vi "T7 Read Cal Constants KAG.vi"(0 "IP:Port":string, 4 "Flash Write Registers":T4(array[cluster])=[{"Register Num"=61800, "Register Name"="INTERNAL_FLASH_KEY", "DataType"="UINT32", "Write Val"=1134709826.0}, {"Register Num"=61810, "Register Name"="INTERNAL_FLASH_READ_POINTER", "DataType"="UINT32", "Write Val"=3948544.0}] {"Write Val" format="%#.0f"}, 5 "Stream Configuration":T2={"Scan Rate (Hz)"=1000.0, "Samples Per Packet"=512, "Resolution Index"=0, "Buffer Size (bytes)"=32768, "NumScans"=1500, "Read Timeout (ms)"=5000, "Scan Table"=[{"Channel"=0, "BipGain"=0, "Input Config"="Single-Ended"}, {"Channel"=1, "BipGain"=0, "Input Config"="Single-Ended"}, {"Channel"=2, "BipGain"=0, "Input Config"="Single-Ended"}, {"Channel"=3, "BipGain"=0, "Input Config"="Single-Ended"}]} {"Samples Per Packet" max=512 step=1; "Buffer Size (bytes)" max=32768 step=1; "Resolution Index" max=8 step=1; "Scan Rate (Hz)" max=100000; "Scan Table"."BipGain" items=["x1", "x10", "x100", "x1000"]; "Scan Table"."Channel" step=1}, 6 "Flash Read Registers":T4(array[cluster])=[{"Register Num"=61812, "Register Name"="INTERNAL_FLASH_READ", "DataType"="UINT32", "Write Val"=0.0}], 7 "Secondary Stream Configurations":T1={"Settling Delay (*5 us)"=0.0, "Clock Source"=0, "Auto Target"=1} {"Auto Target" max=255 step=1; "Clock Source" max=2 step=2; "Settling Delay (*5 us)" min=0 max=5000 step=1}, 11 "error in":errorcluster) -> (8 "Calibration Constants":T5(array[cluster]) {"PSlope" format="%#.13f"; "NSlope" format="%#.13f"; "AvgSlope" format="%#.13f"; "Center" format="%#.13f"; "Offset" format="%#.13f"}, 15 "error out":errorcluster)   [LabVIEW 2022 SP3]
doc: "Write Stream Configuration LabJack Registers via MODBUS. There are a set of registers which comprise the stream configuration registers, and these are written with control values for Scan Rate, NumScans, Resolution, etc. Also, the Scan Table is used to build a Scan List of Stream Configuration Registers which point to streamable AI Channels."
uses:
  T7 Stream Config KAG.ctl
  T7 Secondary Configs KAG.ctl
  T7 Stream Globals KAG.vi
panel:
  in  "Tab Control":T3(tab)=enum."Flash Data"
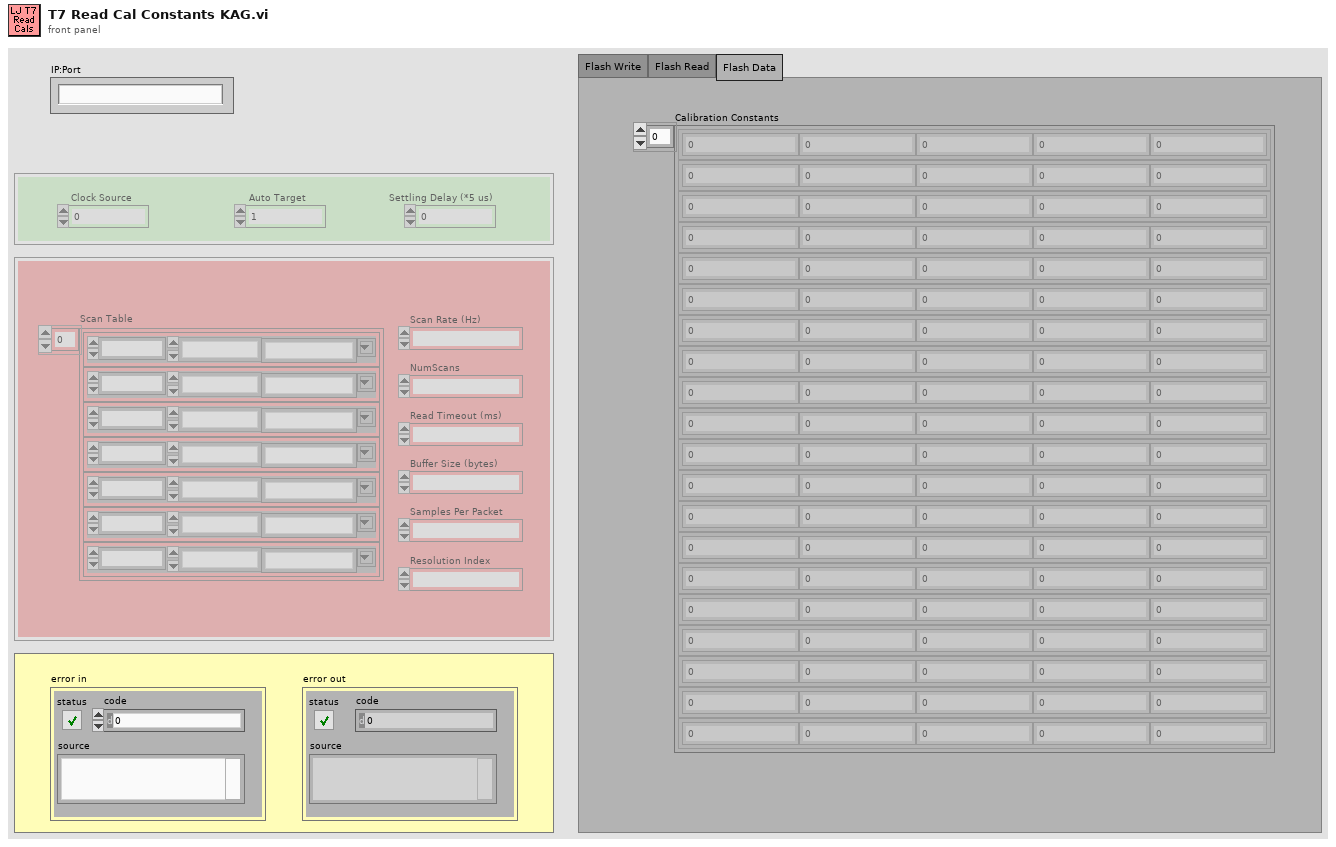
[diagram p1: front panel]
types:
  T1 = typedef "T7 Secondary Configs KAG.ctl" = cluster{"Settling Delay (*5 us)":sgl, "Clock Source":u32, "Auto Target":u32}
  T2 = typedef "T7 Stream Config KAG.ctl" = cluster{"Scan Rate (Hz)":sgl, "Samples Per Packet":u32, "Resolution Index":u32, "Buffer Size (bytes)":u32, "NumScans":u32, "Read Timeout (ms)":u32, "Scan Table":cluster{"Channel":u32, "BipGain":u32, "Input Config":string}[]}
  T3 = enum32{"Flash Write", "Flash Read", "Flash Data"}
  T4 = cluster{"Register Num":i32, "Register Name":string, "DataType":string, "Write Val":dbl}[]
  T5 = cluster{"PSlope":dbl, "NSlope":dbl, "AvgSlope":dbl, "Center":dbl, "Offset":dbl}[]
  T6 = cluster{"Register Num":i32, "Register Name":string, "DataType":string, "Write Val":dbl}
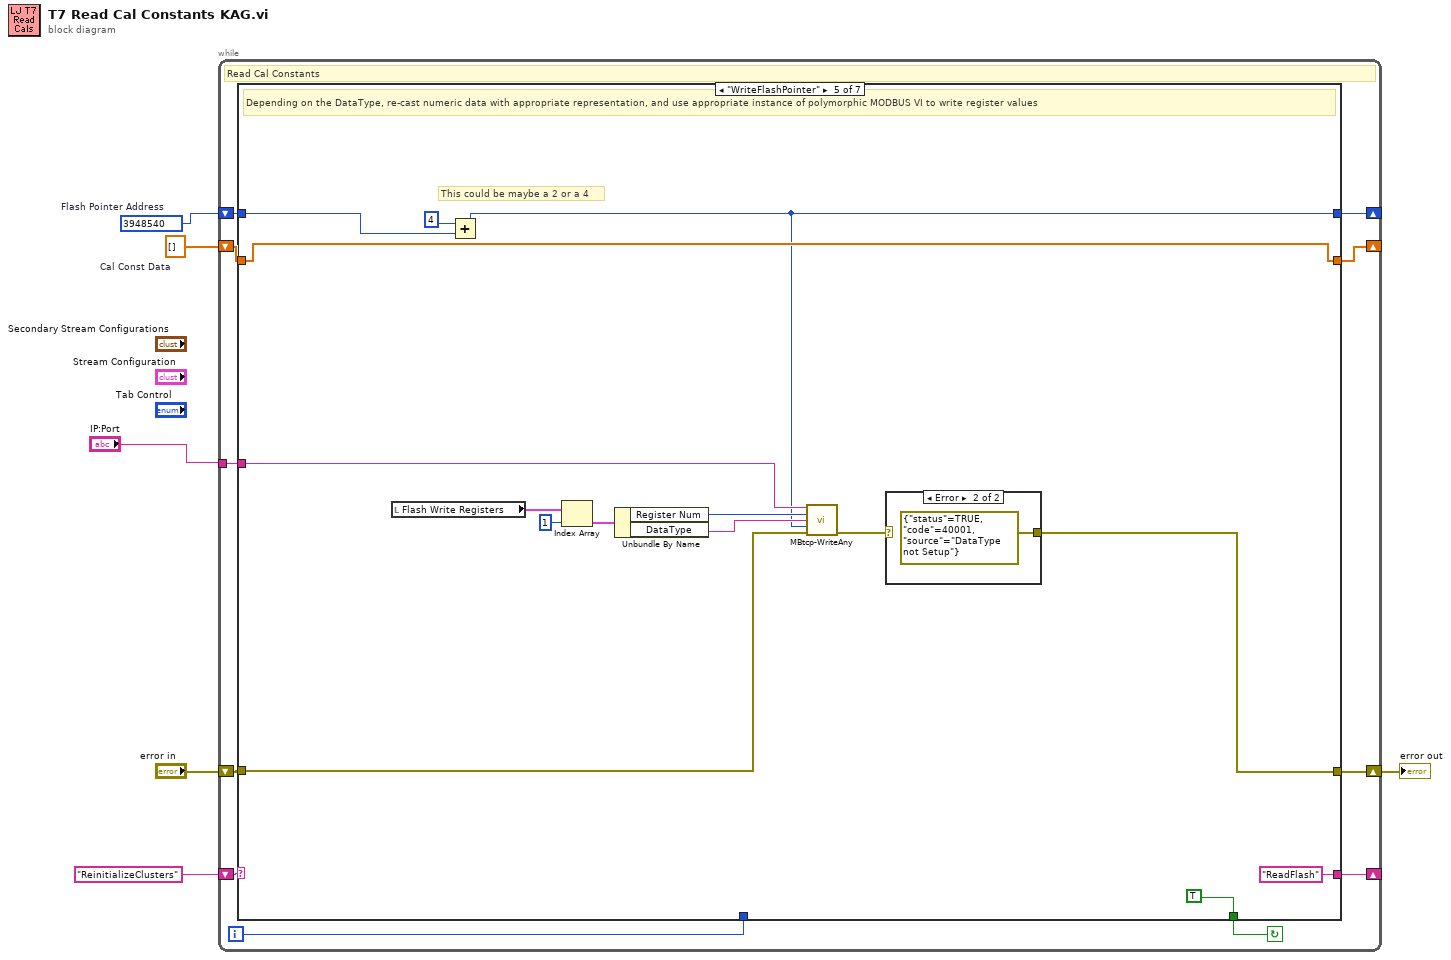
[diagram p0: block diagram]
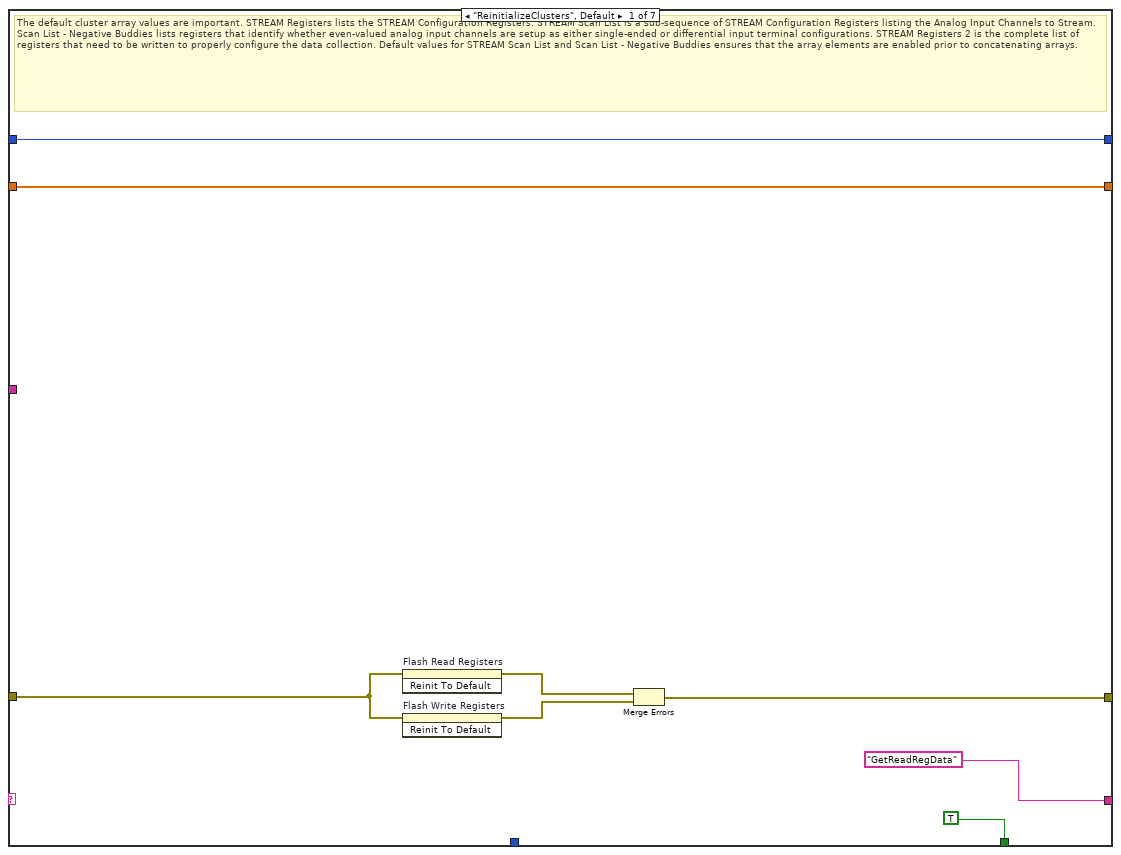
[diagram p2: hidden frame]
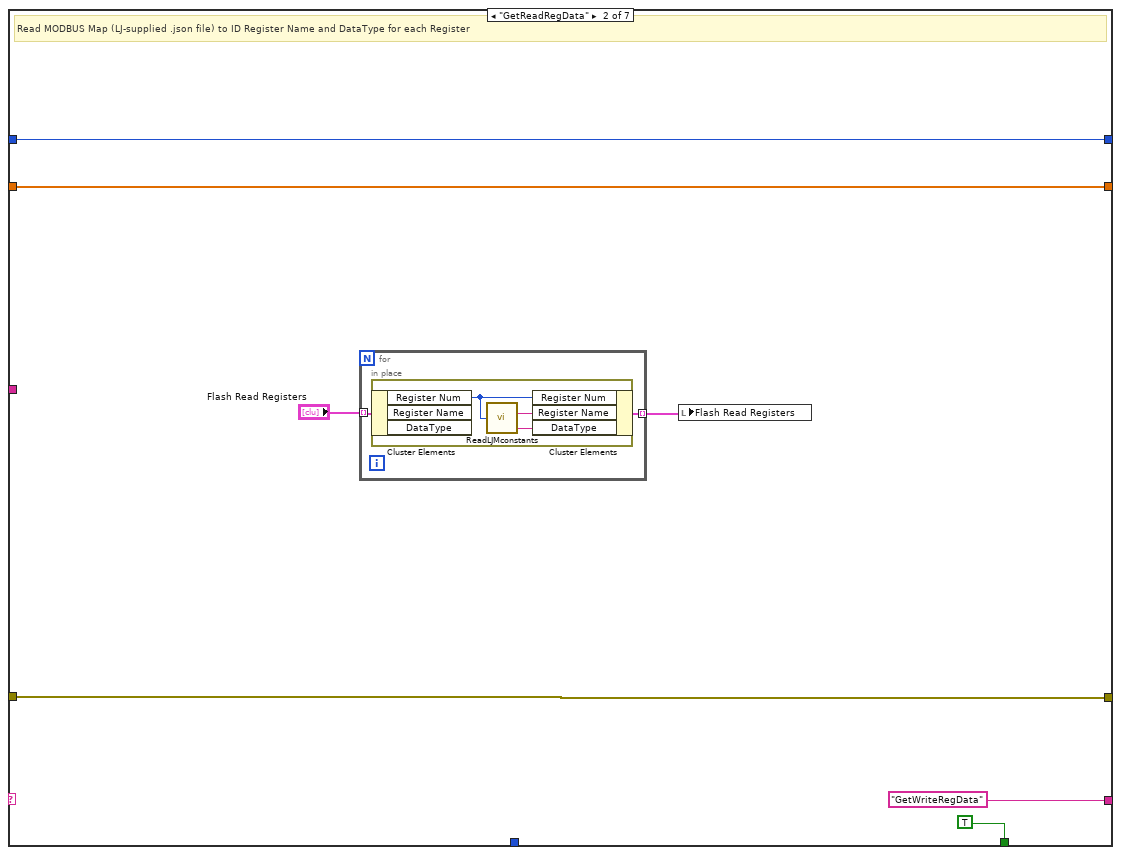
[diagram p3: hidden frame]
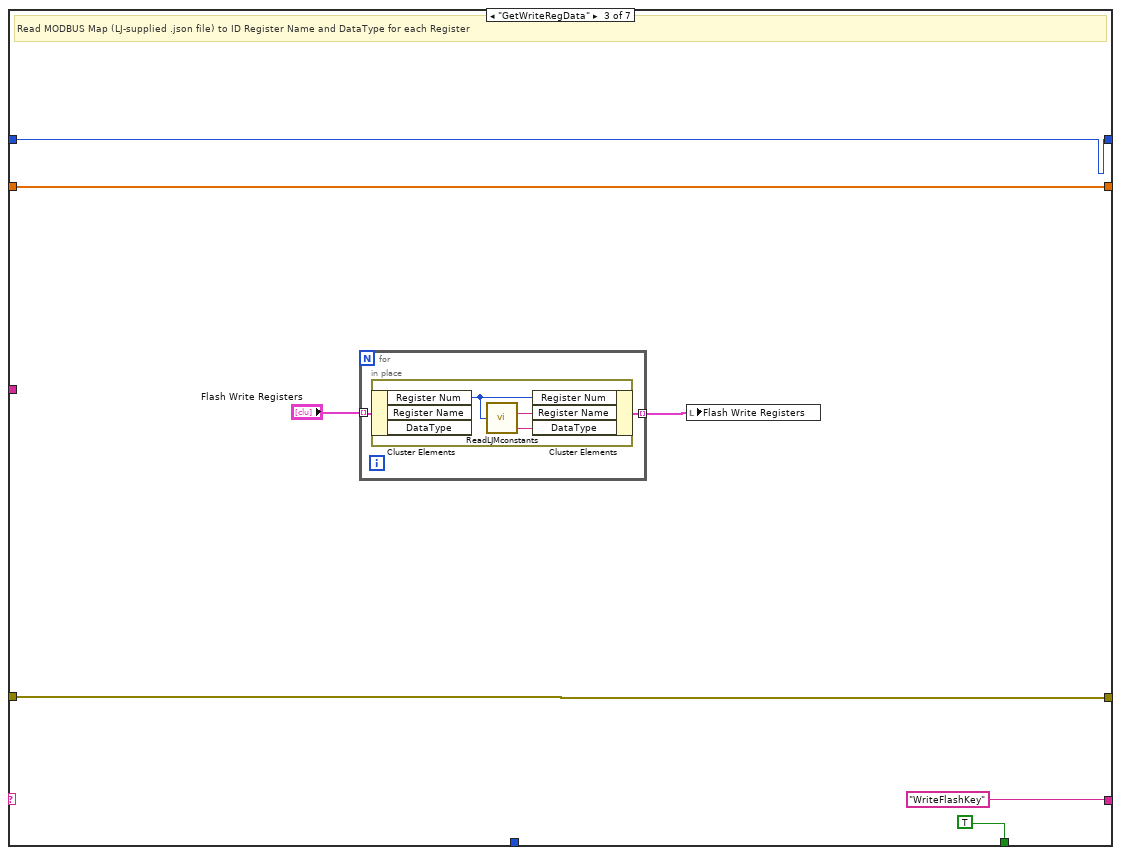
[diagram p4: hidden frame]
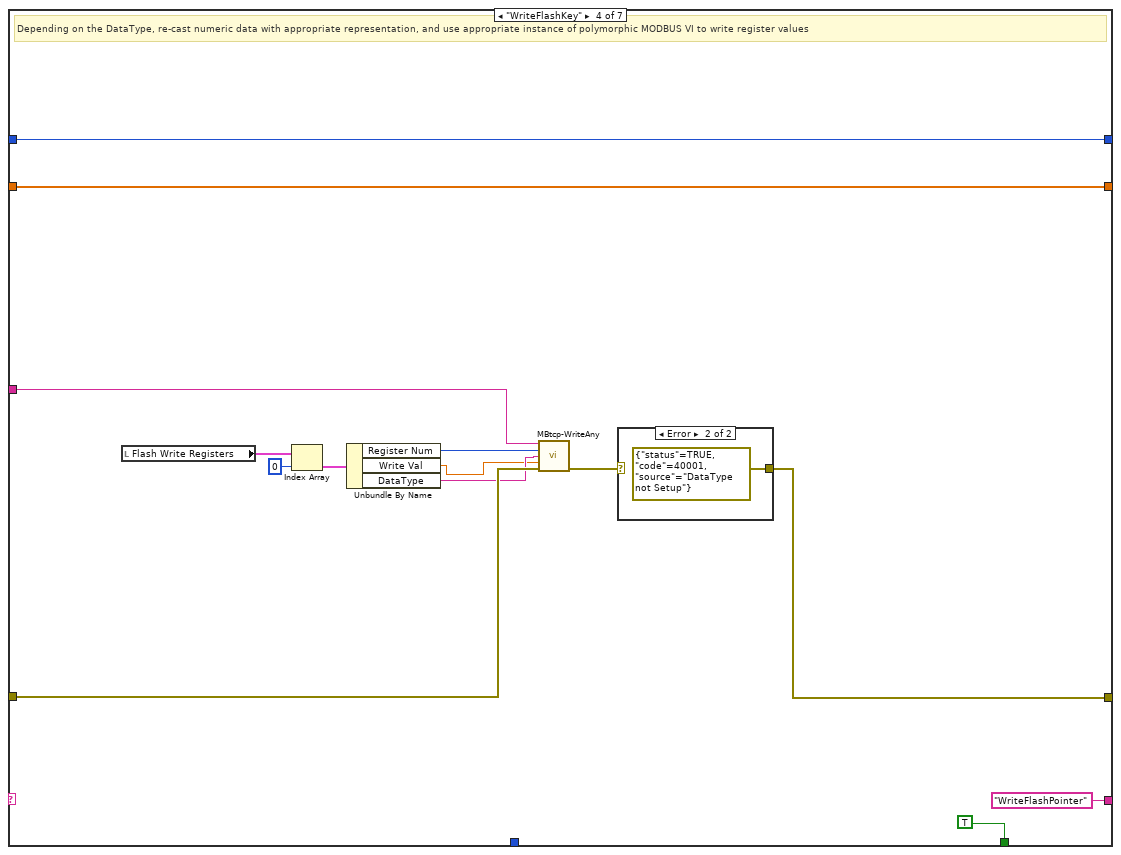
[diagram p5: hidden frame]
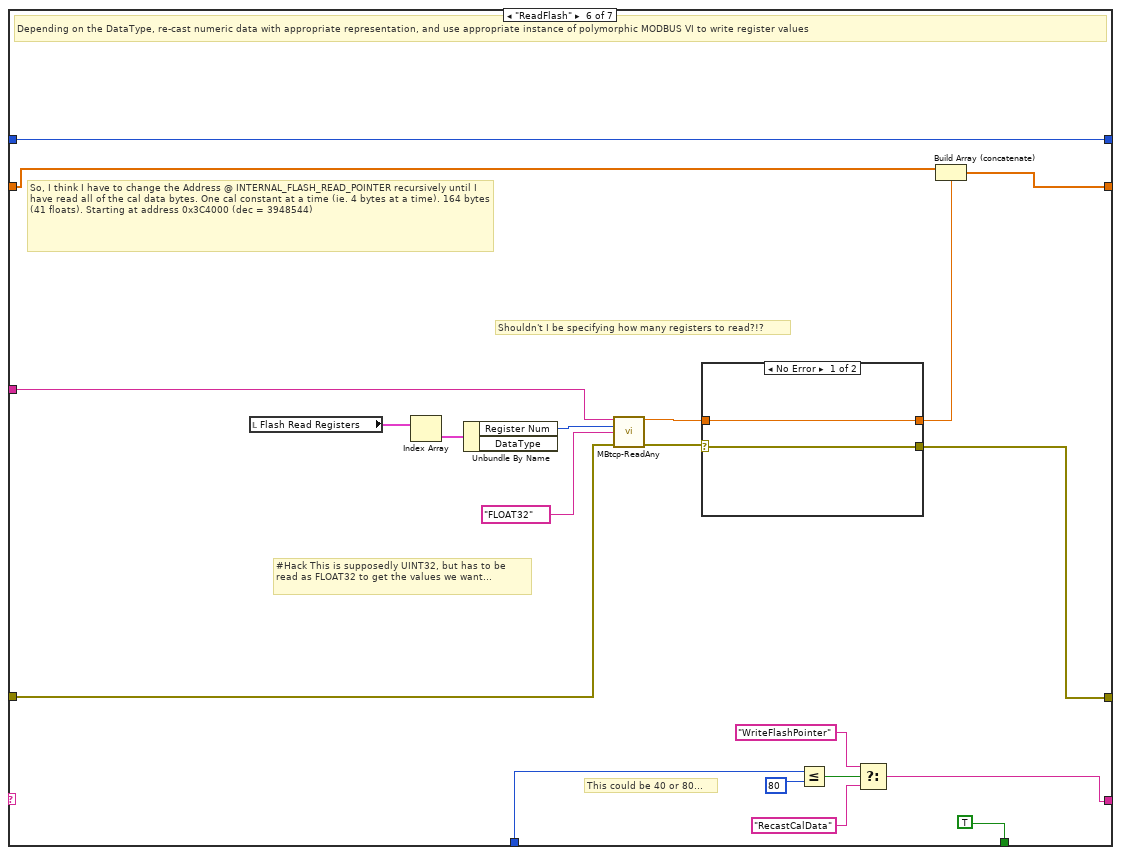
[diagram p8: hidden frame]
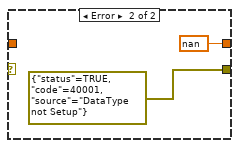
[diagram p9: hidden frame]
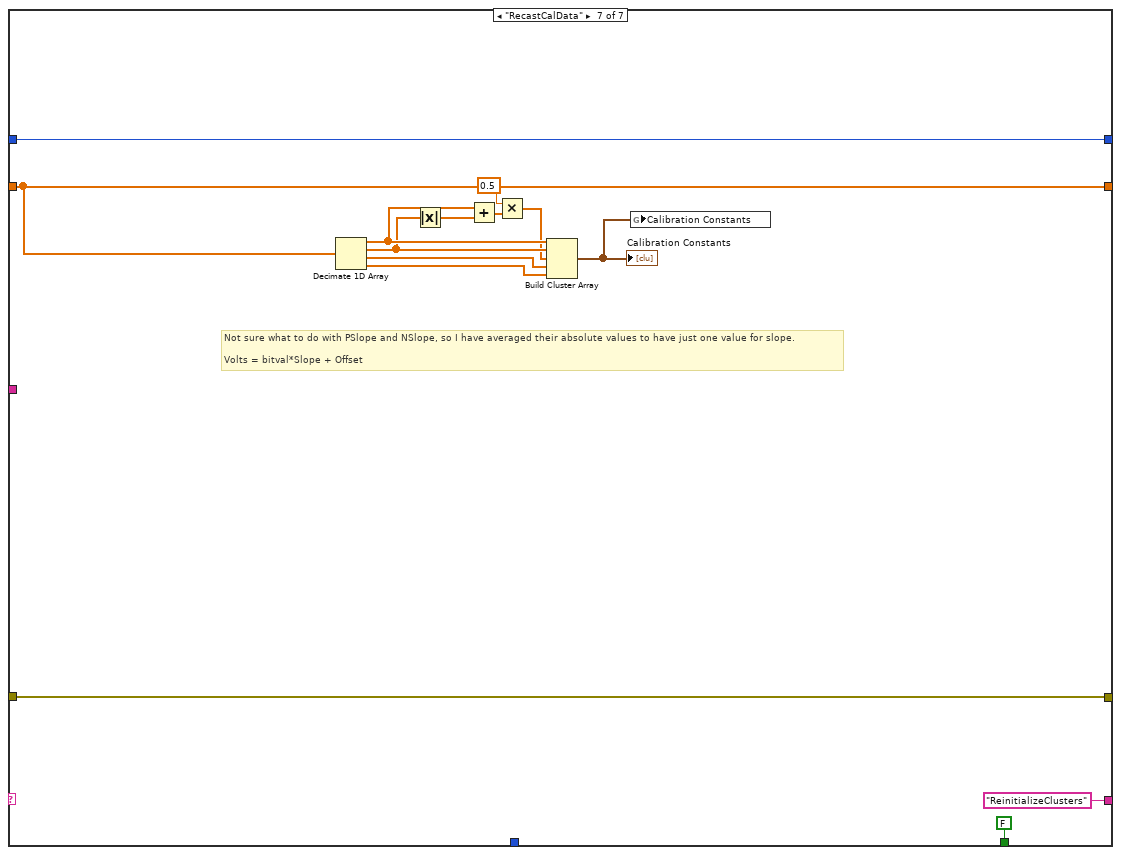
[diagram p10: hidden frame]
diagram:
  w2 = dbl[] []  # Cal Const Data
  w3 = u32 3948540  # Flash Pointer Address
  n1 = while {
    shift-right: [w15] -> _
    shift-left: "ReinitializeClusters" -> [w17]
    shift-right: [w13] -> w4
    shift-left: "error in" -> [w14]
    shift-right: [w7] -> _
    shift-left: w3 -> [w8]
    shift-right: [w11] -> _
    shift-left: w2 -> [w10]
    tunnel: "IP:Port" -> [w9]
    i -> [w12]
    stop <- w16 continue-if-true
    # "Read Cal Constants"
    n2 = case shown="\"WriteFlashPointer\"" w17 {
      tunnel: [TRUE TRUE TRUE TRUE TRUE TRUE FALSE] -> w16
      tunnel: ["GetReadRegData" "GetWriteRegData" "WriteFlashKey" "WriteFlashPointer" "ReadFlash" w92 "ReinitializeClusters"] -> w15
      tunnel: w14 -> [w23 w29 w41 w57 w71 w90 w117]
      tunnel: [w21 w29 w41 w55 w70 w88 w117] -> w13
      tunnel: [w18 w26 w38 w50 w66 w83 w107] -> w7
      tunnel: w12 -> [_ _ _ _ _ w97 _]
      tunnel: [w19 w28 w40 w58 w76 w99 w119] -> w11
      tunnel: w10 -> [w19 w28 w40 w58 w76 w98 w119]
      tunnel: w9 -> [_ _ _ w53 w69 w84 _]
      tunnel: w8 -> [w18 w26 w38 w50 w67 w83 w107]
      frame "ReinitializeClusters", Default {
        # "The default cluster array values are important. STREAM Registers lists the STREAM Configuration Registers. STREAM Scan List is a sub-sequence of STREAM Configuration Registers listing the Analog Input Channels to Stream. Scan List - Negative Buddies lists registers that identify whether even-valued analog input channels are setup as either single-ended or differential input terminal configurations. STREAM Registers 2 is the complete list of registers that need to be written to properly configure the data collection. Default values for STREAM Scan List and Scan List - Negative Buddies ensures that the array elements are enabled prior to concatenating arrays."
        n3 = invoke on="Flash Read Registers" class="Arr (strict)" method="Reinit To Default"(error in=w23) -> (error out=w22:errorcluster)  [unwired: 2 in, 2 out]
        n4 = invoke on="Flash Write Registers" class="Arr (strict)" method="Reinit To Default"(error in=w23) -> (error out=w20:errorcluster)  [unwired: 2 in, 2 out]
        n5 = Merge Errors(w22, w20) -> (w21:errorcluster)
      }
      frame "GetReadRegData" {
        # "Read MODBUS Map (LJ-supplied .json file) to ID Register Name and DataType for each Register"
        n6 = for {
          tunnel: "Flash Read Registers" -> [w34] mode=indexing
          tunnel: [w33] -> w30 mode=indexing
          n7 = in-place {
            n8 = in-place-cluster #1(w34) -> ("Register Num"=w35:i32)  [unwired: 2 out]
            n9 = call "ReadLJMconstants.vi"("Selected Register"=w35) -> ("Register Name"=w37:string, "Data Type"=w36:string)  [unwired: 1 out]
            n10 = in-place-cluster #1("Register Num"=w35, "Register Name"=w37, "DataType"=w36) -> (w33:T6)
          }
        }
        n11 = local write "Flash Read Registers"(w30) -> ()
      }
      frame "GetWriteRegData" {
        # "Read MODBUS Map (LJ-supplied .json file) to ID Register Name and DataType for each Register"
        n12 = for {
          tunnel: "Flash Write Registers" -> [w46] mode=indexing
          tunnel: [w45] -> w42 mode=indexing
          n13 = in-place {
            n14 = in-place-cluster #2(w46) -> ("Register Num"=w47:i32)  [unwired: 2 out]
            n15 = call "ReadLJMconstants.vi"("Selected Register"=w47) -> ("Register Name"=w49:string, "Data Type"=w48:string)  [unwired: 1 out]
            n16 = in-place-cluster #2("Register Num"=w47, "Register Name"=w49, "DataType"=w48) -> (w45:T6)
          }
        }
        n17 = local write "Flash Write Registers"(w42) -> ()
      }
      frame "WriteFlashKey" {
        # "Depending on the DataType, re-cast numeric data with appropriate representation, and use appropriate instance of polymorphic MODBUS VI to write register values"
        n18 = local read "Flash Write Registers"() -> (w61:T4)
        n19 = Index Array(array=w61, index=0) -> (element=w59:T6)
        n20 = Unbundle By Name(w59) -> ("Register Num"=w54:i32, "Write Val"=w51:dbl, "DataType"=w52:string)
        n21 = call "MBtcp-WriteAny.vi"("IP Address"=w53, "Register"=w54, "DataType(:RegisterType)"=w52, "Value to Output"=w51, "Error In"=w57) -> ("error out"=w56:errorcluster)  [unwired: 10 in]
        n22 = case shown="Error" w56 {
          selector: w56 -> [w64 _]
          tunnel: [w64 errorcluster {"status"=TRUE, "code"=40001, "source"="DataType not Setup"} ("error constant")] -> w55
          frame No Error {
          }
          frame Error {
          }
        }
      }
      frame "WriteFlashPointer" {
        # "This could be maybe a 2 or a 4"
        # "Depending on the DataType, re-cast numeric data with appropriate representation, and use appropriate instance of polymorphic MODBUS VI to write register values"
        n23 = local read "Flash Write Registers"() -> (w78:T4)
        n24 = Add(x=u32 4 ("y"), y=w67) -> (x+y=w66:u32)
        n25 = Index Array(array=w78, index=1) -> (element=w72:T6)
        n26 = Unbundle By Name(w72) -> ("Register Num"=w73:i32, "DataType"=w68:string)
        n27 = call "MBtcp-WriteAny.vi"("IP Address"=w69, "Register"=w73, "DataType(:RegisterType)"=w68, "Value to Output"=w66, "Error In"=w71) -> ("error out"=w74:errorcluster)  [unwired: 10 in]
        n28 = case shown="Error" w74 {
          selector: w74 -> [w81 _]
          tunnel: [w81 errorcluster {"status"=TRUE, "code"=40001, "source"="DataType not Setup"} ("error constant")] -> w70
          frame No Error {
          }
          frame Error {
          }
        }
      }
      frame "ReadFlash" {
        # "#Hack This is supposedly UINT32, but has to be read as FLOAT32 to get the values we want..."
        # "This could be 40 or 80..."
        # "Shouldn't I be specifying how many registers to read?!?"
        # "So, I think I have to change the Address @ INTERNAL_FLASH_READ_POINTER recursively until I have read all of the cal data bytes. One cal constant at a time (ie. 4 bytes at a time). 164 bytes (41 floats). Starting at address 0x3C4000 (dec = 3948544)"
        # "Depending on the DataType, re-cast numeric data with appropriate representation, and use appropriate instance of polymorphic MODBUS VI to write register values"
        n29 = local read "Flash Read Registers"() -> (w101:T4)
        n30 = Index Array(array=w101) -> (element=w100:T6)  [unwired: 1 in]
        n31 = Unbundle By Name(w100) -> ("Register Num"=w91:i32)  [unwired: 1 out]
        n32 = call "MBtcp-ReadAny.vi"("IP Address"=w84, "Register"=w91, "DataType(:RegisterType)"="FLOAT32" ("Data type"), "Error In"=w90) -> ("Value"=w86:dbl, "error out"=w87:errorcluster)  [unwired: 9 in, 1 out]
        n33 = case shown="No Error" w87 {
          selector: w87 -> [w104 _]
          tunnel: [w103 nan] -> w89
          tunnel: [w104 errorcluster {"status"=TRUE, "code"=40001, "source"="DataType not Setup"} ("error constant")] -> w88
          tunnel: w86 -> [w103 _]
          frame No Error {
          }
          frame Error {
          }
        }
        n34 = Less Or Equal?(x=w97, y=80) -> (x <= y?=w95:bool)
        n35 = Select(t="WriteFlashPointer", s=w95, f="RecastCalData") -> (s? t:f=w92:string)
        n36 = Build Array (concatenate)(w98, w89) -> (w99:dbl[])
      }
      frame "RecastCalData" {
        # "Not sure what to do with PSlope and NSlope, so I have averaged their absolute values to have just one value for slope.\n\nVolts = bitval*Slope + Offset"
        n37 = Decimate 1D Array(w119) -> (w116:dbl[], w115:dbl[], w111:dbl[], w110:dbl[])
        n38 = Absolute Value(x=w115) -> (abs(x)=w109:dbl[])
        n39 = Add(x=w116, y=w109) -> (x+y=w114:dbl[])
        n40 = Multiply(x=0.5, y=w114) -> (x*y=w112:dbl[])
        n41 = Build Cluster Array(w116, w115, w112, w111, w110) -> (w108:cluster{dbl, dbl, dbl, dbl, dbl}[])
        "Calibration Constants" <- w108
        n42 = global write "T7 Stream Globals KAG.vi" "Calibration Constants"(w108) -> ()
      }
    }
  }
  "error out" <- w4
